vi "Find Average Center.vi"(5 "Position":i32, 7 "Tray Number":i32, 8 "Assembly Type":string, 9 "XYZTheta":dbl[](array[numeric]), 11 "Gantry In":refnum<k24>) -> (1 "XYZTheta":dbl[](array[numeric]) format="%.6g", 3 "Gantry Out":refnum<k24>)   [LabVIEW 2021, in "Component Tray.lvclass"]
uses:
  Component Tray.lvclass
  Find Component.ctl
  Controller/Camera/Machine Vision.ctl
  C:/Program Files (x86)/Aerotech/A3200/LabVIEW/2010/Bin/Aerotech.A3200.dll
  Program Files (x86)/Aerotech/A3200/LabVIEW/2010/Bin/Aerotech.A3200.dll
  Controller/Camera/Image processing.ctl
  Controller/Camera/Camera settings.ctl
  Controller/Camera/Material.ctl
  Controller/Camera/Edmund Optics/Edmund Optics.lvclass
  C:/Users/HEP/Documents/GitHub/Gantry/UCSB-Gantry-HEP-main/Classes/Controller/Camera/Camera.lvclass
  Controller/Camera/Camera.lvclass
  Controller/Motion/A3200/A3200.lvclass
  Controller/Motion/Motion.lvclass
  Routine/TypeOfHexaboard.ctl
  Routine/Routine.lvclass
panel:
  out "Current Z High Speed":dbl
  out "Current XY High Speed":dbl
  out "current Z low speed":dbl
  out "current XY speed":dbl
  in  "Z high":dbl=12.5
  in  "XY high":dbl=50.0
  in  "Z low":dbl=0.05
  in  "XY low":dbl=0.1
  in  "Predict fiducials":bool
  out "Low Speed":bool
  out "X":bool
  out "Y":bool
  out "Z":bool
  out "High Speed":bool
  in  "Go to CH191/FD5":bool
  in  "Go to CH197/FD4":bool
  out "Program Stopped":bool
  out "XY Graph":cluster{"X":dbl, "Y":dbl}[](graph)
  out "Sensor ID Location":dbl[](array[numeric])
  in  "Go to Sensor ID":bool
  out "CH1 Location":dbl[](array[numeric])
  in  "Verify CH1":bool
  out "CH1 correct?":bool
  in  "Go to CH1":bool
  in  "Focus step size":dbl format="%#_13g"
  in  "number of focus steps":i32
  out "Average Strength":dbl
  in  "Focus":bool
  in  "Material":T1
  out "All fiducials recorded":bool
  in  "Override presets":bool
  in  "Camera settings":T2={"Gamma"=1.6, "Gain"=0, "Sharpness"=0, "Contrast"=0.0, "Exposure"=0.0078125} {"Exposure" min=0.000244140625 max=0.5 scale=0.0002..0.5; "Contrast" min=0.0 max=1.0 scale=0.001..1.0; "Sharpness" min=0 max=2 step=1 scale=0.0..2.0; "Gain" min=0 max=100 step=1 scale=0.1..100.0; "Gamma" min=0.01 max=10.0 scale=0.01..10.0}
  in  "Image processing":T3={"Brightness"=128.0, "Contrast"=45.0, "Gamma"=1.0471123} {"Brightness" scale=0.0..400.0; "Contrast" scale=0.0..90.0; "Gamma" scale=0.005..5.0}
  in  "Machine Vision":T4=enum."Sensor Fiducials"
  out "Gantry":dbl[](array[numeric]) format="%.6g"
  out "Sum":dbl[](array[numeric]) format="%.6g"
  out "CH197/FD4 XY":dbl[](array[numeric]) format="%.6g"
  out "CH8/FD2 XY":dbl[](array[numeric]) format="%.6g"
  out "CH191/FD5 XY":dbl[](array[numeric]) format="%.6g"
  out "CH1/FD1 XY":dbl[](array[numeric]) format="%.6g"
  in  "Record CH8/FD2":bool
  in  "Record CH197/FD4":bool
  in  "Record CH191/FD5":bool
  in  "Record CH1/FD1":bool
  in  "Go to CH8/FD2":bool
  in  "Go to CH1/FD1":bool
  in  "Joystick":bool
  out "Camera":dbl[](array[numeric]) format="%.6g"
  in  "Go to Center":bool
  in  "Component":T5
  in  "Stop Program":bool
  out "Image":T6(plugin-control)
  # "Requires CH1/FD1 found."
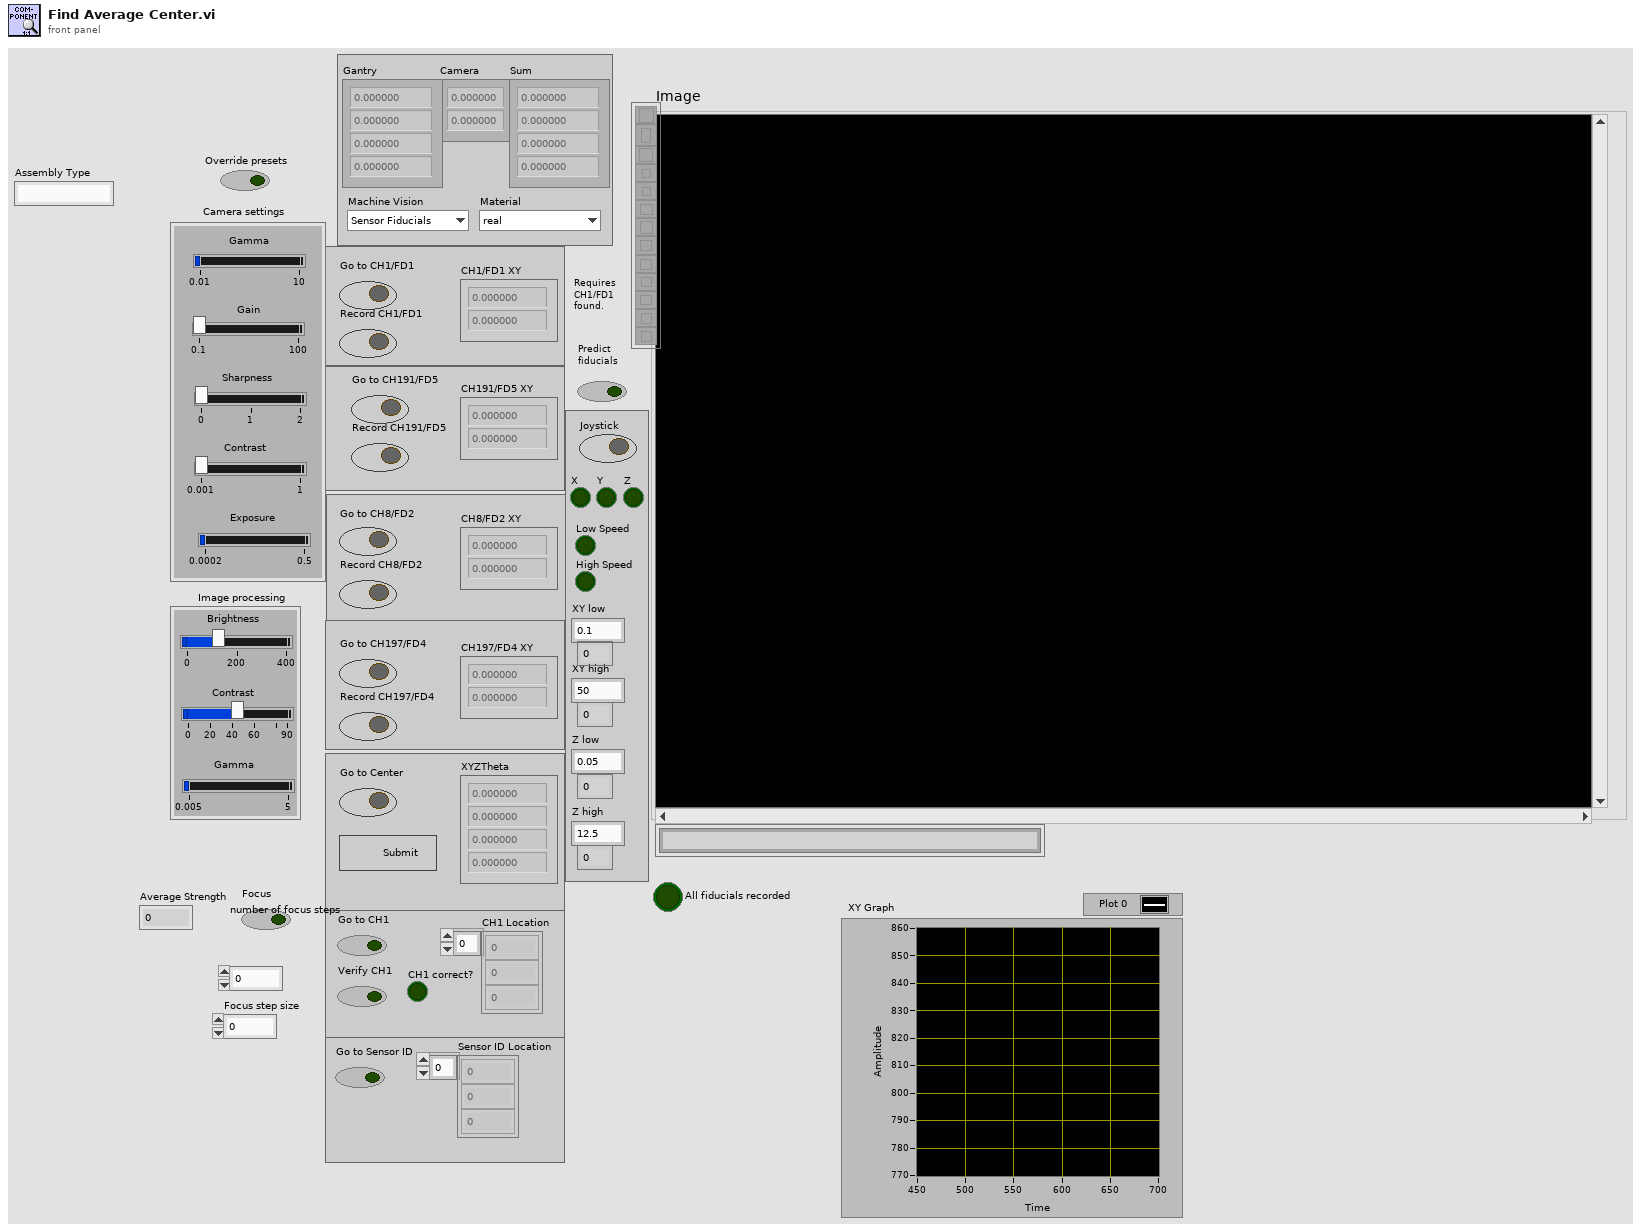
[diagram p1: front panel]
types:
  T1 = typedef "Camera.lvclass/Material.ctl" = enum16{"real", "dummy", "PETG"}
  T2 = typedef "Camera.lvclass/Camera settings.ctl" = cluster{"Gamma":dbl, "Gain":i64, "Sharpness":i64, "Contrast":dbl, "Exposure":dbl}
  T3 = typedef "Camera.lvclass/Image processing.ctl" = cluster{"Brightness":sgl, "Contrast":sgl, "Gamma":sgl}
  T4 = typedef "Camera.lvclass/Machine Vision.ctl" = enum16{"None", "Tray Fiducials", "Sensor Fiducials", "HPK Silicon", "Partial Hexaboard", "Partial Hexaboard Test", "100um dot", "Hexaboard", "Corner (TL, BR)", "Corner (BL, TR)", "V3 Sensor Cross", "V3 Sensor Circle", "test"}
  T5 = typedef "Component Tray.lvclass/Find Component.ctl" = cluster{"New Fiducials":dbl[], "Past Fiducials":dbl[][], "XYZTheta":dbl[], "Fiducials Path":path, "Position":i32, "CH1 Location":dbl[], "Sensor ID Location":dbl[]}
  T6 = typedef "IMAQ Image.ctl" = refnum<image>
  T7 = typedef "Routine.lvclass/TypeOfHexaboard.ctl" = enum16{"Full Sensor", "Full PCB", "Right Partial PCB", "Right Partial Sensor", "Al Dummy Right Partial Sensor"}
  T8 = typedef "File Paths.ctl" = cluster{"Glue Pattern Folder":path, "Carrier Tray Folder":path, "Pick Up Tool Fixture Folder":path, "Components Folder":path, "Bellows Tool Offset.txt":path, "Pick Up Tool Offset.txt":path, "Dispense Tip Offset.txt":path, "Log Files":path, "Gantry Assembly Map.txt":path, "Syringe and offset map.txt":path, "Controllers Folder":path, "Local dbase config":path}
  T9 = enum8{"Enabled", "Disabled", "Disabled and Grayed Out"}
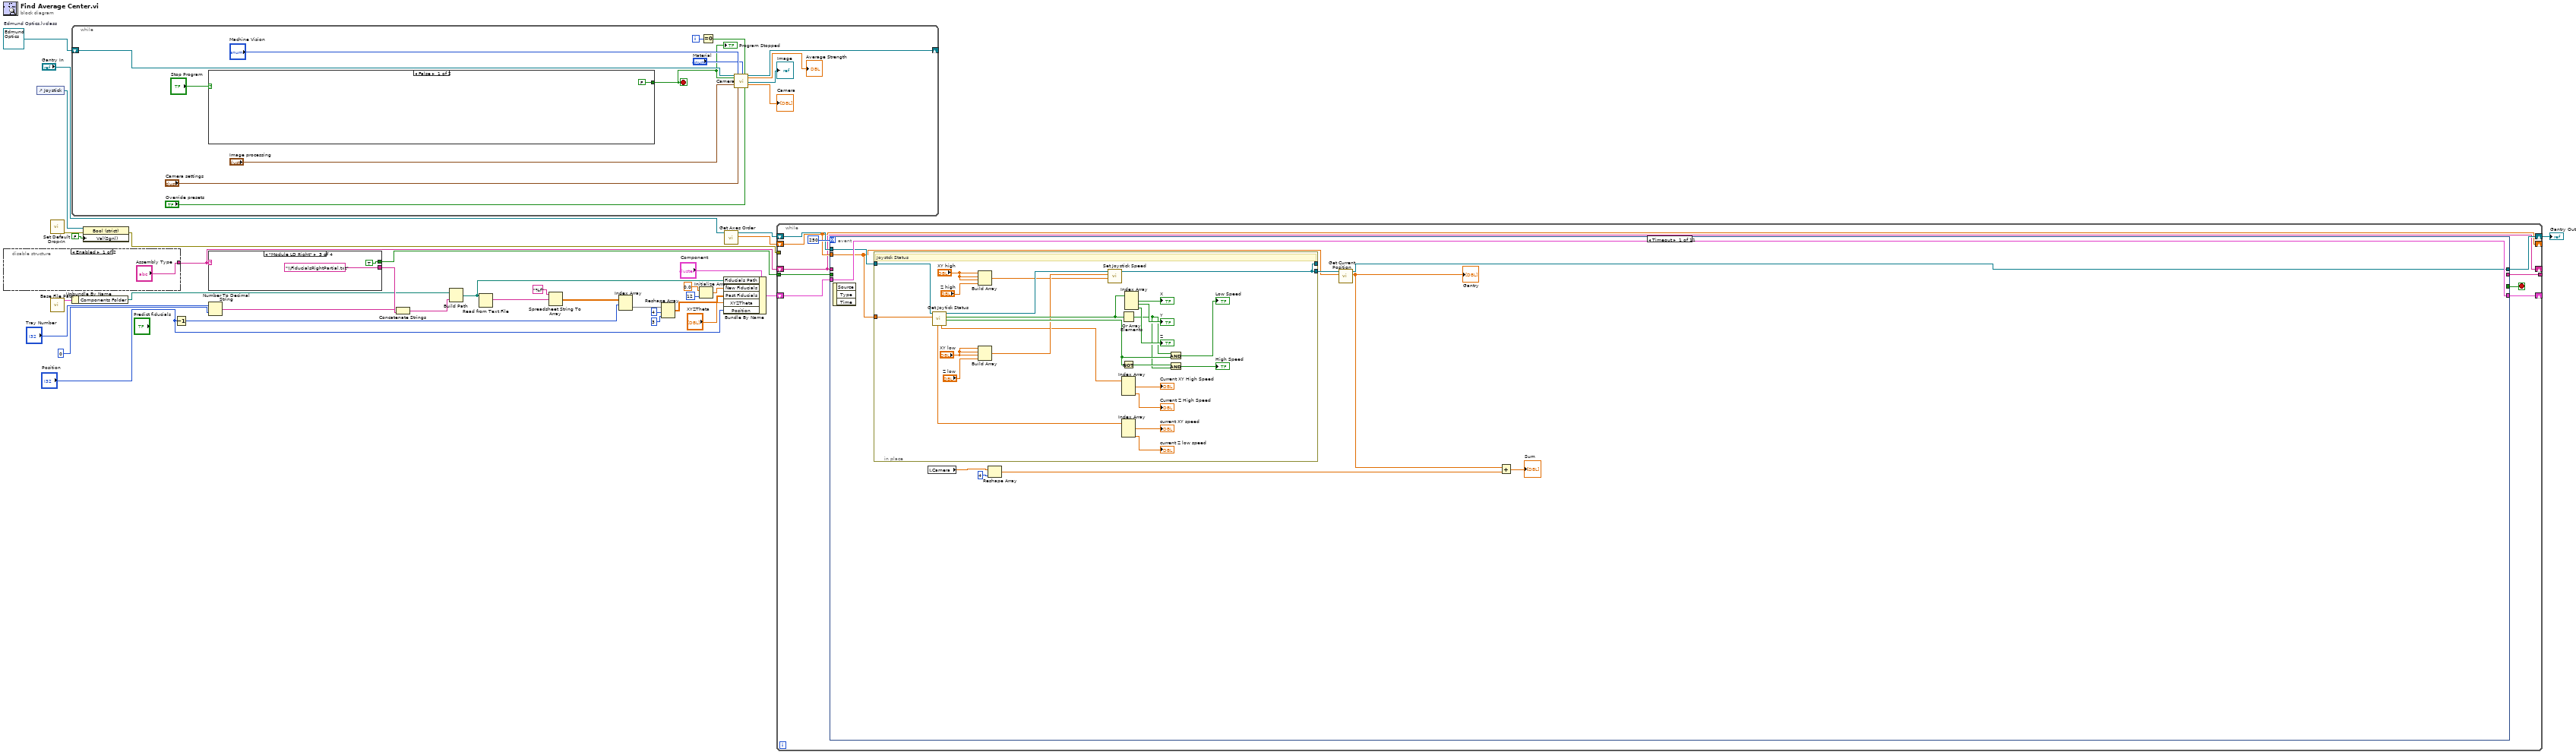
[diagram p0: block diagram]
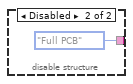
[diagram p2: hidden frame]
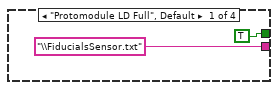
[diagram p3: hidden frame]
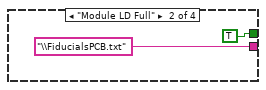
[diagram p4: hidden frame]
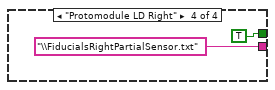
[diagram p5: hidden frame]
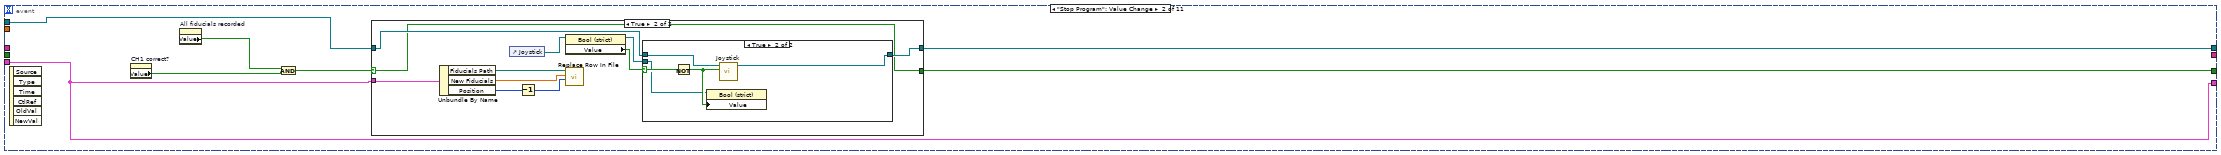
[diagram p6: hidden frame]
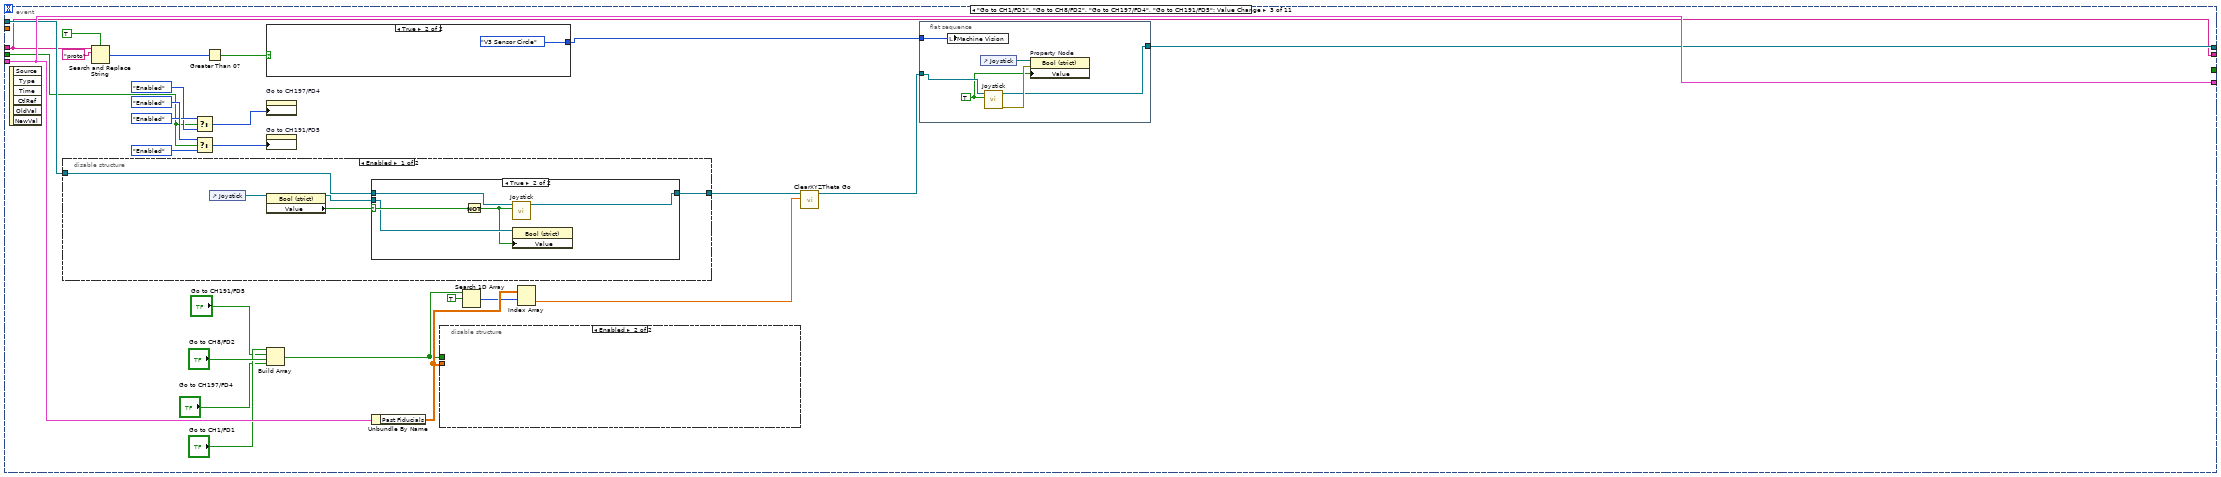
[diagram p9: hidden frame]
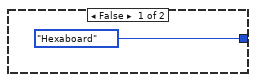
[diagram p10: hidden frame]
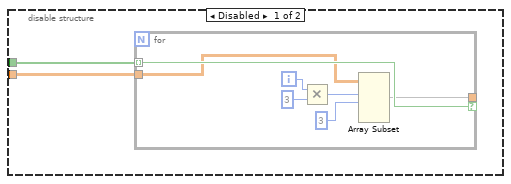
[diagram p11: hidden frame]
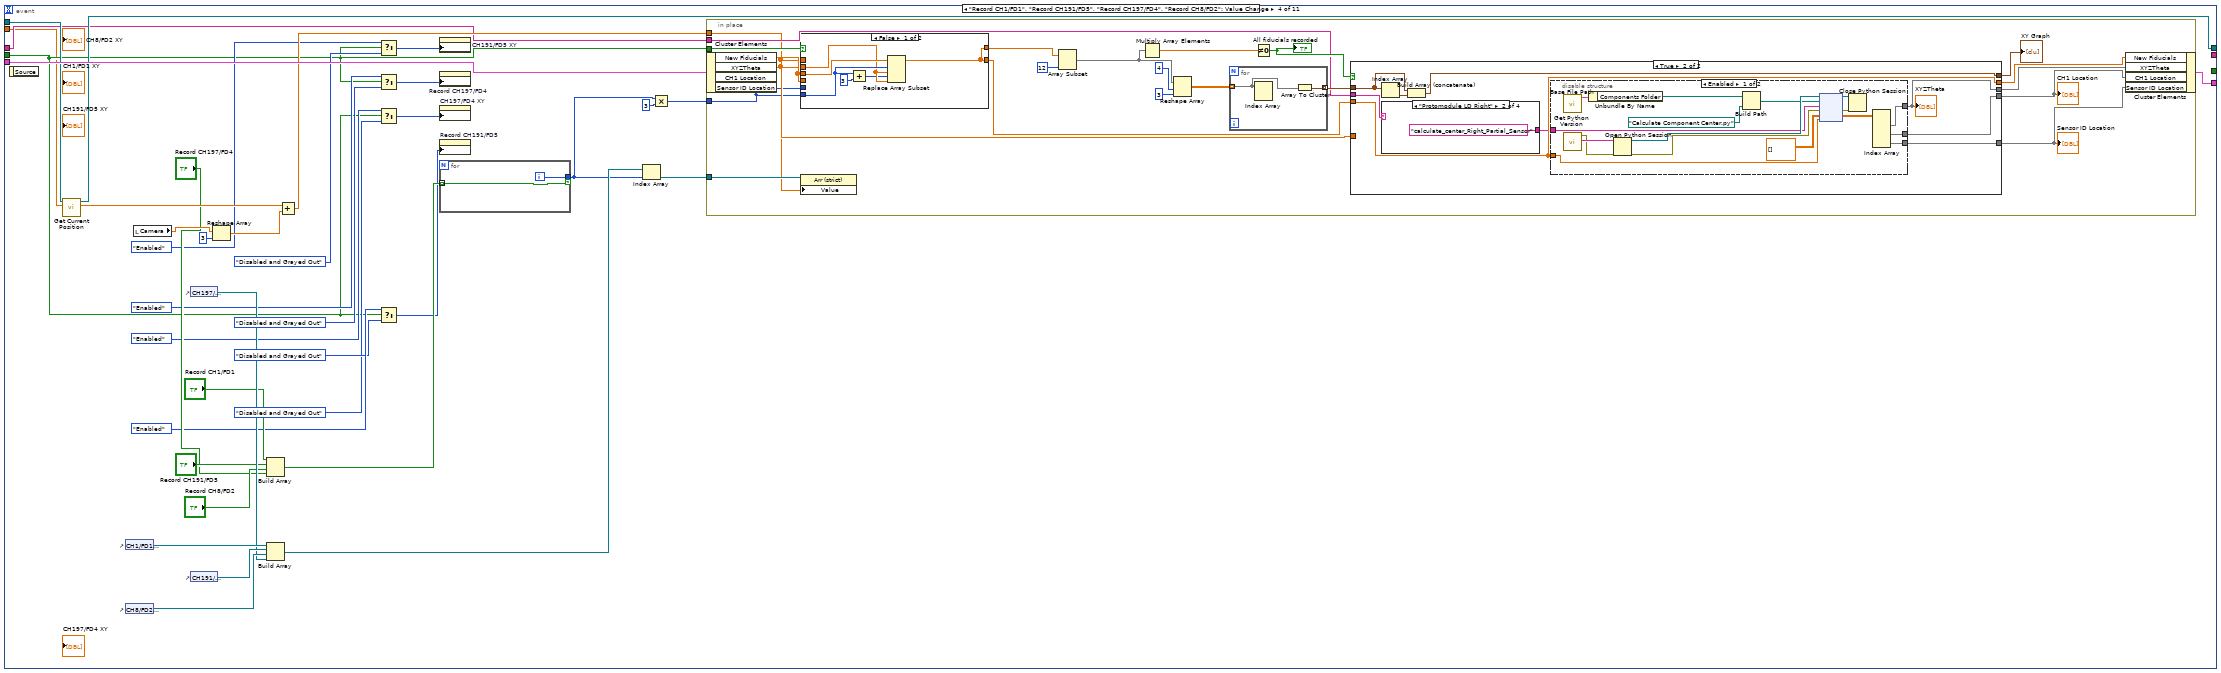
[diagram p14: hidden frame]
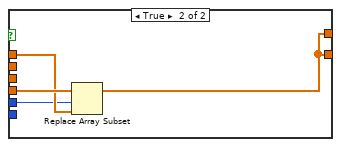
[diagram p15: hidden frame]
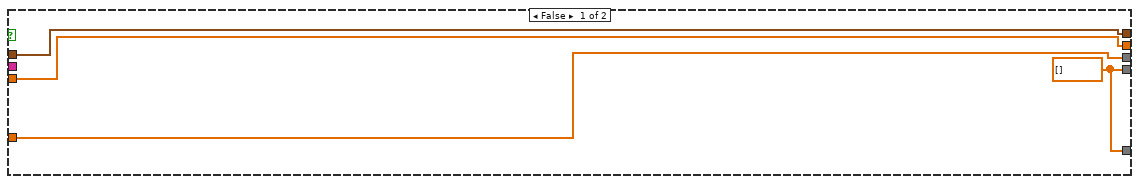
[diagram p16: hidden frame]
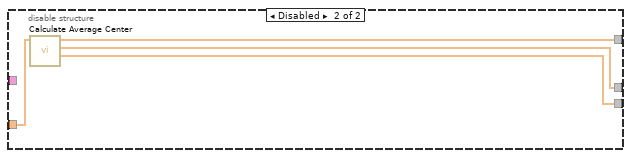
[diagram p17: hidden frame]
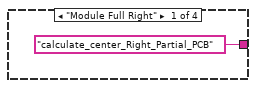
[diagram p18: hidden frame]
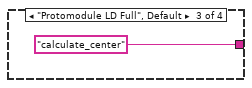
[diagram p19: hidden frame]
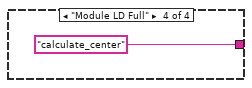
[diagram p20: hidden frame]
diagram:
  w30 = refnum<class "Edmund Optics.lvclass"> refnum  # Edmund Optics.lvclass
  n1 = disable-structure shown="Enabled" {
    disable-tunnel: ["Assembly Type" TypeOfHexaboard."Full PCB" ("Type of Hexaboard")] -> w9
    frame Enabled {
    }
    frame Disabled {
    }
  }
  n2 = control-ref of="Joystick"() -> (w33:refnum<vi>)
  n3 = call "Set Default Drop-In.vi"() -> ("error out"=w12:errorcluster)  [unwired: 11 in]
  n4 = call "Base File Path.vi"() -> ("Paths Out"=w21:T8)  [unwired: 11 in]
  n5 = while {
    shift-right: [w46] -> _
    shift-left: w30 -> [w50]
    i -> [w42]
    stop <- w37 stop-if-true
    n6 = case shown="False" "Stop Program" {
      tunnel: [FALSE w52] -> w37
      frame False {
      }
      frame True {
        n7 = property on="CH1 correct?" class="Bool (strict)"() -> ("Value"=w53:bool)  [unwired: 2 in, 2 out]
        n8 = property on="All fiducials recorded" class="Bool (strict)"() -> ("Value"=w55:bool)  [unwired: 2 in, 2 out]
        n9 = And(x=w55, y=w53) -> (x .and. y?=w54:bool)
        n10 = case shown="False" w54 {
          tunnel: [FALSE TRUE] -> w52
          frame False {
            n11 = One Button Dialog(message="At least one fiducial not recorded or component orientation not verified.") -> ()  [unwired: 1 in, 1 out]
          }
          frame True {
            n12 = property on="All fiducials recorded" class="Bool (strict)"("Val(Sgnl)"=FALSE) -> ()  [unwired: 2 in, 2 out]
          }
        }
      }
    }
    "Program Stopped" <- w37
    n13 = Equal To 0?(x=w42) -> (x = 0?=w41:bool)
    n14 = call "Camera.vi"("Camera in"=w50, "Stop"=w37, "BCG Image Processing"="Image processing", "Machine Vision"="Machine Vision", "Camera settings"="Camera settings", "Material"="Material", "Loop 0"=w41, "Override presets"="Override presets") -> ("Camera out"=w46:refnum<class "Edmund Optics.lvclass">, "Average Strength"=→"Average Strength":dbl, "Image"=→"Image":T6, "Camera"=→"Camera":dbl[])  [unwired: 5 in, 3 out]
  }
  n15 = Unbundle By Name(w21) -> ("Components Folder"=w23:path)
  n16 = property class="Bool (strict)"(reference=w33, error in=w12, "Val(Sgnl)"=FALSE) -> (error out=w31:errorcluster)  [unwired: 1 out]
  n17 = Decrement(x="Position") -> (x-1=w13:i32)
  n18 = case shown="\"Module LD Right\"" w9 {
    tunnel: ["\\FiducialsSensor.txt" ("string") "\\FiducialsPCB.txt" ("string") "\\FiducialsRightPartial.txt" ("string") "\\FiducialsRightPartialSensor.txt" ("string")] -> w25
    tunnel: [TRUE TRUE TRUE TRUE] -> w8
    frame "Protomodule LD Full", Default {
    }
    frame "Module LD Full" {
    }
    frame "Module LD Right" {
    }
    frame "Protomodule LD Right" {
    }
  }
  n19 = Number To Decimal String(number="Tray Number", width (-)=i16 0) -> (decimal integer string=w24:string)
  n20 = Concatenate Strings "Concatenate Strings"(w24, w25) -> (w26:string)
  n21 = Build Path(base path=w23, name or relative path=w26) -> (appended path=w16:path)
  n22 = Read from Text File(file (use dialog)=w16) -> (text=w27:string)  [unwired: 3 in, 3 out]
  n23 = Spreadsheet String To Array(format string="%f", spreadsheet string=w27) -> (array=w29:dbl[][])  [unwired: 2 in]
  n24 = Index Array "Index Array"(array=w29, index (row)=w13) -> (element=w4:dbl[])  [unwired: 1 in]
  n25 = Reshape Array(w4, 4 ("dimension size"), 3 ("dimension size")) -> (w1:dbl[][])
  n26 = Initialize Array(0.0 ("element"), 12 ("dimension size")) -> (w19:dbl[])
  n27 = Bundle By Name "Bundle By Name"(cluster="Component", "Fiducials Path"=w16, "New Fiducials"=w19, "Past Fiducials"=w1, "XYZTheta"="XYZTheta", "Position"="Position") -> (w10:T5)
  n28 = call "Get Axes Order.vi"("Gantry In"="Gantry In") -> ("Axes Order"=w5:dbl[], "Gantry Out"=w6:refnum<k24>)  [unwired: 8 in, 1 out]
  n29 = while {
    shift-right: [w75] -> _
    shift-left: w10 -> [w76]
    tunnel: w31 -> [_]
    shift-right: [w72] -> w11
    shift-left: w6 -> [w73]
    tunnel: [w71] -> _
    tunnel: w8 -> [w70]
    shift-right: [w69] -> _
    shift-left: w5 -> [w69]
    shift-right: [w68] -> _
    shift-left: w9 -> [w68]
    stop <- w77 stop-if-true
    n30 = event shown="[0] Timeout" {
      selector: _ -> [_ _ _ _ _ _ _ _ _ _ _]
      dyn-events: _ -> [_ _ _ _ _ _ _ _ _ _ _]
      timeout: 250 -> [_ _ _ _ _ _ _ _ _ _ _]
      tunnel: [_ w116 _ _ _ _ _ _ _ _ _] -> w77
      tunnel: w76 -> [w86 w118 w165 w231 w317 w355 w403 w410 w425 w440 w450]
      tunnel: [w86 w118 w165 w230 w316 w355 w403 w410 w425 w440 w450] -> w75
      tunnel: w73 -> [w80 w119 w164 w222 w315 w357 w402 w406 w421 w436 w451]
      tunnel: [w82 w117 w161 w220 w315 w356 w400 w404 w419 w434 w451] -> w72
      tunnel: w68 -> [_ _ w141 w219 w311 _ _ _ _ _ _]
      tunnel: [_ _ w141 _ _ _ _ _ _ _ _] -> w71
      tunnel: w70 -> [_ _ w150 w195 _ _ _ _ _ _ _]
      tunnel: w69 -> [w78 _ _ w194 _ w345 _ _ _ _ _]
      event Timeout {
        n31 = event-data() -> ()  [unwired: 1 in, 3 out]
        n32 = in-place {
          in-place-border: w80 -> [w112]
          in-place-border: [w100] -> _
          in-place-border: w78 -> [w111]
          in-place-border: [w100] -> w79
          # "Joystck Status"
          n33 = call "Get Joytick Status.vi"("Axes Order"=w111, "Gantry In"=w112) -> ("JoystickLowSpeedActive"=w105:bool, "Joystick Status"=w107:bool[], "Gantry Out"=w101:refnum<k24>, "High Speeds"=w89:dbl[], "Low Speeds"=w88:dbl[])  [unwired: 4 in, 1 out]
          n34 = Build Array("XY high", "XY high", "XY high", "Z high") -> (w94:dbl[])
          n35 = Build Array("XY low", "XY low", "XY low", "Z low") -> (w95:dbl[])
          n36 = call "Set Joystick Speed.vi"("High Speed Inputs"=w94, "Low Speed Inputs"=w95, "Gantry"=w101) -> ("Controller Out"=w100:refnum<k24>)  [unwired: 7 in, 1 out]
          n37 = Or Array Elements(Boolean array=w107) -> (logical OR=w103:bool)
          n38 = Not(x=w105) -> (.not. x?=w104:bool)
          n39 = Index Array(array=w89) -> (element #1=→"Current XY High Speed":dbl, element #3=→"Current Z High Speed":dbl)  [unwired: 3 in, 1 out]
          n40 = Index Array(array=w88) -> (element #1=→"current XY speed":dbl, element #3=→"current Z low speed":dbl)  [unwired: 3 in, 1 out]
          n41 = Index Array(array=w107) -> (element #1=→"X":bool, element #2=→"Y":bool, element #3=→"Z":bool)  [unwired: 3 in]
          n42 = And(x=w103, y=w105) -> (x .and. y?=→"Low Speed":bool)
          n43 = And(x=w104, y=w103) -> (x .and. y?=→"High Speed":bool)
        }
        n44 = local read "Camera"() -> (w85:dbl[])
        n45 = Reshape Array(w85, 4 ("dimension size")) -> (w83:dbl[])
        n46 = call "Get Current Position.vi"("Axes Order"=w78, "Gantry In"=w79) -> ("XYZTheta Out"=w81:dbl[], "Gantry Out"=w82:refnum<k24>)  [unwired: 7 in, 1 out]
        "Gantry" <- w81
        n47 = Add(x=w81, y=w83) -> (x+y=→"Sum":dbl[])
      }
      event "Stop Program": Value Change {
        n48 = event-data() -> ()  [unwired: 1 in, 6 out]
        n49 = property on="CH1 correct?" class="Bool (strict)"() -> ("Value"=w115:bool)  [unwired: 2 in, 2 out]
        n50 = property on="All fiducials recorded" class="Bool (strict)"() -> ("Value"=w114:bool)  [unwired: 2 in, 2 out]
        n51 = And(x=w114, y=w115) -> (x .and. y?=w113:bool)
        n52 = case shown="True" w113 {
          selector: w113 -> [w120 w129]
          tunnel: w119 -> [w121 w131]
          tunnel: w118 -> [_ w132]
          tunnel: [w121 w130] -> w117
          tunnel: [w120 w129] -> w116
          frame False {
          }
          frame True {
            n53 = Unbundle By Name(w132) -> ("Fiducials Path"=w126:path, "New Fiducials"=w125:dbl[], "Position"=w127:i32)
            n54 = control-ref of="Joystick"() -> (w123:refnum<vi>)
            n55 = Decrement(x=w127) -> (x-1=w128:i32)
            n56 = property class="Bool (strict)"(reference=w123) -> (reference out=w122:refnum<vi>, "Value"=w124:bool)  [unwired: 1 in, 1 out]
            n57 = call "Replace Row In File.vi"("Index"=w128, "Insert Array"=w125, "Path"=w126) -> ()  [unwired: 8 in, 1 out]
            n58 = case shown="True" w124 {
              selector: w124 -> [_ w138]
              tunnel: w131 -> [w133 w137]
              tunnel: [w133 w136] -> w130
              tunnel: w122 -> [_ w134]
              frame False {
              }
              frame True {
                n59 = Not(x=w138) -> (.not. x?=w135:bool)
                n60 = property class="Bool (strict)"(reference=w134, "Value"=w135) -> ()  [unwired: 1 in, 2 out]
                n61 = call "Joystick.vi"("Joystick"=w135, "Gantry In"=w137) -> ("Gantry Out"=w136:refnum<k24>)  [unwired: 8 in, 1 out]
              }
            }
          }
        }
      }
      event "Go to CH1/FD1", "Go to CH8/FD2", "Go to CH197/FD4", "Go to CH191/FD5": Value Change {
        n62 = event-data() -> ()  [unwired: 1 in, 6 out]
        n63 = disable-structure shown="Enabled" {
          disable-tunnel: w164 -> [w179 _]
          disable-tunnel: [w178 _] -> w163
          frame Enabled {
            n64 = control-ref of="Joystick"() -> (w177:refnum<vi>)
            n65 = property class="Bool (strict)"(reference=w177) -> (reference out=w180:refnum<vi>, "Value"=w181:bool)  [unwired: 1 in, 1 out]
            n66 = case shown="True" w181 {
              selector: w181 -> [_ w187]
              tunnel: w179 -> [w182 w185]
              tunnel: [w182 w183] -> w178
              tunnel: w180 -> [_ w186]
              frame False {
              }
              frame True {
                n67 = Not(x=w187) -> (.not. x?=w184:bool)
                n68 = call "Joystick.vi"("Joystick"=w184, "Gantry In"=w185) -> ("Gantry Out"=w183:refnum<k24>)  [unwired: 8 in, 1 out]
                n69 = property class="Bool (strict)"(reference=w186, "Value"=w184) -> ()  [unwired: 1 in, 2 out]
              }
            }
          }
          frame Disabled {
          }
        }
        n70 = Search and Replace String(case sensitive?=TRUE ("ignore case? (F)"), input string=w141, search string="proto") -> (number of replacements=w142:i32)  [unwired: 5 in, 3 out]
        n71 = Select(t=T9."Enabled" ("Disabled"), s=w150, f=T9."Enabled" ("Disabled")) -> (s? t:f=w151:T9)
        n72 = Select(t=T9."Enabled" ("Disabled"), s=w150, f=T9."Enabled" ("Disabled")) -> (s? t:f=w154:T9)
        n73 = Greater Than 0?(x=w142) -> (x > 0?=w139:bool)
        n74 = case shown="True" w139 {
          tunnel: [Machine_Vision."Hexaboard" ("Machine Vision") Machine_Vision."V3 Sensor Circle" ("Machine Vision")] -> w140
          frame False {
          }
          frame True {
          }
        }
        n75 = property on="Go to CH197/FD4" class="Bool"("DisabledEnum"=w151) -> ()  [unwired: 2 in, 2 out]
        n76 = property on="Go to CH191/FD5" class="Bool"("DisabledEnum"=w154) -> ()  [unwired: 2 in, 2 out]
        n77 = Build Array "Build Array"("Go to CH1/FD1", "Go to CH191/FD5", "Go to CH8/FD2", "Go to CH197/FD4") -> (w147:bool[])
        n78 = Unbundle By Name(w165) -> ("Past Fiducials"=w149:dbl[][])
        n79 = disable-structure shown="Enabled" {
          disable-tunnel: w149 -> [w169 _]
          disable-tunnel: w147 -> [w168 _]
          frame Disabled {
            n80 = for {
              tunnel: w168 -> [w176] mode=indexing
              tunnel: w169 -> [w175]
              tunnel: [w170] -> _ if=w176
              i -> [w173]
              n81 = Multiply(x=w173, y=3) -> (x*y=w171:i32)
              n82 = Array Subset "Array Subset"(array=w175, index (row)=w171, length (row)=3 ("length")) -> (w170:dbl[][])  [unwired: 2 in]
            }
          }
          frame Enabled {
          }
        }
        n83 = Search 1D Array(1D array=w147, element=TRUE) -> (index of element=w145:i32)  [unwired: 1 in]
        n84 = Index Array(array=w149, index (row)=w145) -> (element=w148:dbl[])  [unwired: 1 in]
        n85 = call "ClearXYZTheta Go.vi"("XYZTheta In"=w148, "Gantry In"=w163) -> ("Gantry Out"=w162:refnum<k24>)  [unwired: 7 in, 2 out]
        n86 = flat-sequence {
          tunnel: w162 -> [w193]
          tunnel: [w190] -> w161
          tunnel: w140 -> [w188]
          frame #0 {
            w189 = TRUE
            n87 = local write "Machine Vision"(w188) -> ()
            n88 = control-ref of="Joystick"() -> (w192:refnum<vi>)
            n89 = call "Joystick.vi"("Joystick"=w189, "Gantry In"=w193) -> ("error out"=w191:errorcluster, "Gantry Out"=w190:refnum<k24>)  [unwired: 8 in]
            n90 = property on="Property Node" class="Bool (strict)"(reference=w192, error in=w191, "Value"=w189) -> ()  [unwired: 2 out]
          }
        }
      }
      event "Record CH1/FD1", "Record CH191/FD5", "Record CH197/FD4", "Record CH8/FD2": Value Change {
        n91 = event-data() -> ()  [unwired: 1 in, 1 out]
        n92 = call "Get Current Position.vi"("Axes Order"=w194, "Gantry In"=w222) -> ("XYZTheta Out"=w221:dbl[], "Gantry Out"=w220:refnum<k24>)  [unwired: 7 in, 1 out]
        n93 = control-ref of="CH1/FD1 XY"() -> (w217:refnum<vi>)
        n94 = control-ref of="CH8/FD2 XY"() -> (w215:refnum<vi>)
        n95 = local read "Camera"() -> (w225:dbl[])
        n96 = control-ref of="CH197/FD4 XY"() -> (w214:refnum<vi>)
        n97 = control-ref of="CH191/FD5 XY"() -> (w216:refnum<vi>)
        n98 = Reshape Array(w225, 3 ("dimension size")) -> (w224:dbl[])
        n99 = Build Array "Build Array"("Record CH1/FD1", "Record CH191/FD5", "Record CH8/FD2", "Record CH197/FD4") -> (w218:bool[])
        n100 = Build Array "Build Array"(w217, w216, w215, w214) -> (w229:refnum<vi>[])
        n101 = Add(x=w221, y=w224) -> (x+y=w223:dbl[])
        n102 = Select(t=T9."Enabled" ("Disabled"), s=w195, f=T9."Disabled and Grayed Out" ("Disabled")) -> (s? t:f=w200:T9)
        n103 = Select(t=T9."Enabled" ("Disabled"), s=w195, f=T9."Disabled and Grayed Out") -> (s? t:f=w204:T9)
        n104 = Select(t=T9."Enabled" ("Disabled"), s=w195, f=T9."Disabled and Grayed Out" ("Disabled")) -> (s? t:f=w196:T9)
        n105 = Select(t=T9."Enabled" ("Disabled"), s=w195, f=T9."Disabled and Grayed Out") -> (s? t:f=w206:T9)
        n106 = property on="CH191/FD5 XY" class="Arr (strict)"("DisabledEnum"=w200) -> ()  [unwired: 2 in, 2 out]
        n107 = property on="Record CH197/FD4" class="Bool"("DisabledEnum"=w204) -> ()  [unwired: 2 in, 2 out]
        n108 = property on="CH197/FD4 XY" class="Arr (strict)"("DisabledEnum"=w196) -> ()  [unwired: 2 in, 2 out]
        n109 = property on="Record CH191/FD5" class="Bool"("DisabledEnum"=w206) -> ()  [unwired: 2 in, 2 out]
        n110 = for {
          tunnel: w218 -> [w232] mode=indexing
          tunnel: [w233] -> w209 if=w232
          i -> [w233]
        }
        n111 = Index Array "Index Array"(array=w229, index=w209) -> (element=w228:refnum<vi>)
        n112 = Multiply(x=w209, y=3) -> (x*y=w226:i32)
        n113 = in-place {
          in-place-border: w226 -> [w235]
          in-place-border: w228 -> [w253]
          in-place-border: w223 -> [w236]
          in-place-border: w219 -> [w240]
          in-place-border: w195 -> [w238]
          n114 = in-place-cluster #1(w231) -> ("New Fiducials"=w237:dbl[], "XYZTheta"=w252:dbl[])  [unwired: 2 out]
          n115 = case shown="False" w238 {
            tunnel: w237 -> [w261 _]
            tunnel: w235 -> [w260 _]
            tunnel: w236 -> [w259 _]
            tunnel: [w256 w262] -> w239
            tunnel: w237 -> [_ w265]
            tunnel: w236 -> [_ w264]
            tunnel: w235 -> [_ w263]
            tunnel: [w256 w262] -> w234
            frame False {
              n116 = Add(x=w260, y=3) -> (x+y=w257:i32)
              n117 = Replace Array Subset "Replace Array Subset"(array=w261, new element #1=w259, index #1=w260, new element #2=w259, index #2=w257) -> (w256:dbl[])
            }
            frame True {
              n118 = Replace Array Subset "Replace Array Subset"(array=w265, new element=w264, index=w263) -> (w262:dbl[])
            }
          }
          n119 = property class="Arr (strict)"(reference=w253, "Value"=w236) -> ()  [unwired: 1 in, 2 out]
          n120 = Array Subset "Array Subset"(array=w234, length=12) -> (w247:dbl[])  [unwired: 1 in]
          n121 = Multiply Array Elements(1:w247) -> (0:w250:dbl)
          n122 = Reshape Array "Reshape Array"(w247, 4 ("dimension size"), 3 ("dimension size")) -> (w244:dbl[][])
          n123 = for {
            tunnel: w244 -> [w266] mode=indexing
            tunnel: [w267] -> w243 mode=indexing
            n124 = Index Array(array=w266) -> ()  [unwired: 2 in, 2 out]
            n125 = Array To Cluster(array=w266) -> (cluster=w267:cluster{"[0]":dbl, "[1]":dbl})
          }
          n126 = Not Equal To 0?(x=w250) -> (x != 0?=w241:bool)
          "All fiducials recorded" <- w241
          n127 = case shown="True" w241 {
            tunnel: [w270 w273] -> w255
            tunnel: w239 -> [w271 w277]
            tunnel: [w271 w277] -> w254
            tunnel: w252 -> [w270 _]
            tunnel: [w269 w274] -> w249
            tunnel: [w269 w275] -> w248
            tunnel: w243 -> [w268 w280]
            tunnel: [w268 w278] -> w242
            tunnel: w240 -> [_ w276]
            frame False {
              w269 = dbl[] [] ("CH1 location")
            }
            frame True {
              n128 = Index Array(array=w280) -> (element=w279:cluster{"[0]":dbl, "[1]":dbl})  [unwired: 1 in]
              n129 = case shown="\"Protomodule LD Right\"" w276 {
                tunnel: ["calculate_center_Right_Partial_PCB" ("function name") "calculate_center_Right_Partial_Sensor" ("function name") "calculate_center" ("function name") "calculate_center" ("function name")] -> w272
                frame "Module Full Right" {
                }
                frame "Protomodule LD Right" {
                }
                frame "Protomodule LD Full", Default {
                }
                frame "Module LD Full" {
                }
              }
              n130 = Build Array (concatenate)(w280, w279) -> (w278:cluster{"[0]":dbl, "[1]":dbl}[])
              n131 = disable-structure shown="Enabled" {
                disable-tunnel: w277 -> [w288 w298]
                disable-tunnel: [w284 w301] -> w275
                disable-tunnel: [w285 w300] -> w274
                disable-tunnel: [w286 w299] -> w273
                disable-tunnel: w272 -> [w283 _]
                frame Enabled {
                  n132 = call "Base File Path.vi"() -> ("Paths Out"=w293:T8)  [unwired: 11 in]
                  n133 = call "Get Python Version.vi"() -> ("Python Version"=w282:string, "error out"=w281:errorcluster)  [unwired: 10 in]
                  n134 = Unbundle By Name(w293) -> ("Components Folder"=w291:path)
                  n135 = Open Python Session(python version=w282, 3:w281) -> (session out=w297:refnum<k35>, error out=w295:errorcluster)  [unwired: 1 in]
                  n136 = Build Path(base path=w291, name or relative path=path "Calculate Component Center.py") -> (appended path=w290:path)
                  n137 = node(w297, w290, w283, w295, dbl[][] [], w288) -> (w296:refnum<k35>, w294:errorcluster, w287:dbl[][])  [unwired: 1 in, 2 out]
                  n138 = Close Python Session(session in=w296, error in=w294) -> ()  [unwired: 1 out]
                  n139 = Index Array(array=w287) -> (element #1=w286:dbl[], element #2=w285:dbl[], element #3=w284:dbl[])  [unwired: 6 in]
                }
                frame Disabled {
                  n140 = call "Calculate Average Center.vi"("Gantry Fiducials"=w298) -> ("Sensor ID Location"=w301:dbl[], "CH1 Location"=w300:dbl[], "XYZTheta"=w299:dbl[])  [unwired: 8 in]
                }
              }
              "XYZTheta" <- w273
            }
          }
          "CH1 Location" <- w249
          "Sensor ID Location" <- w248
          "XY Graph" <- w242
          n141 = in-place-cluster #1("New Fiducials"=w254, "XYZTheta"=w255, "CH1 Location"=w249, "Sensor ID Location"=w248) -> (w230:T5)
        }
      }
      event "Predict fiducials": Value Change {
        n142 = event-data() -> ()  [unwired: 1 in, 6 out]
        n143 = Unbundle By Name(w317) -> ("New Fiducials"=w336:dbl[], "Position"=w332:i32)  [unwired: 1 out]
        n144 = Search and Replace String(case sensitive?=TRUE ("ignore case? (F)"), input string=w311, search string="proto") -> (number of replacements=w308:i32)  [unwired: 5 in, 3 out]
        n145 = Reshape Array(w336, 4 ("dimension size"), 3 ("dimension size")) -> (w333:dbl[][])
        n146 = Greater Than 0?(x=w308) -> (x > 0?=w307:bool)
        n147 = case shown="False" w307 {
          tunnel: [dbl[] [-160.0, 70.0] ("x") dbl[] [-165.98, 75.999] ("x")] -> w306
          frame False {
          }
          frame True {
          }
        }
        n148 = Equal?(x=w332, y=1) -> (x = y?=w330:bool)
        n149 = case shown="False" w330 {
          tunnel: w306 -> [w342 w344]
          tunnel: [w342 w343] -> w329
          frame False {
          }
          frame True {
            n150 = Negate(x=w344) -> (-x=w343:dbl[])
          }
        }
        n151 = Index Array(array=w329) -> (element #1=w324:dbl, element #2=w323:dbl)  [unwired: 2 in]
        n152 = Build Array(w324, 0.0 ("element"), 0.0 ("element")) -> (w325:dbl[])
        n153 = Build Array(w324, w323, 0.0 ("element")) -> (w322:dbl[])
        n154 = Build Array(0.0 ("element"), w323, 0.0 ("element")) -> (w326:dbl[])
        n155 = Build Array(w325, w326, w322) -> (w321:dbl[][])
        n156 = Index Array(array=w333) -> (element=w320:dbl[])  [unwired: 2 in]
        n157 = for {
          tunnel: w321 -> [w341] mode=indexing
          tunnel: w320 -> [w340]
          tunnel: [w339] -> w319 mode=indexing
          n158 = Add(x=w341, y=w340) -> (x+y=w339:dbl[])
        }
        n159 = Build Array (concatenate)(w320, w319) -> (w318:dbl[][])
        n160 = Bundle By Name(cluster=w317, "Past Fiducials"=w318) -> (w316:T5)
      }
      event "Focus": Value Change {
        n161 = event-data() -> ()  [unwired: 1 in, 6 out]
        n162 = Divide(x="number of focus steps", y=2) -> (x/y=w360:dbl)
        n163 = Multiply(x=w360, y="Focus step size") -> (x*y=w358:dbl)
        n164 = call "Joystick.vi"("Joystick"=FALSE, "Gantry In"=w357) -> ("Gantry Out"=w351:refnum<k24>)  [unwired: 8 in, 1 out]
        n165 = Negate(x=w358) -> (-x=w352:dbl)
        n166 = call "Z Go.vi"("Increment"=TRUE, "Return Immediately"=FALSE ("Increment"), "Speed In"=1.0 ("Speed"), "Position In"=w352, "Gantry In"=w351) -> ("error out"=w349:errorcluster, "Gantry Out"=w350:refnum<k24>)  [unwired: 3 in, 2 out]
        n167 = for {
          N: "number of focus steps" -> [_]
          tunnel: [w378] -> w371 mode=indexing
          tunnel: w349 -> [w377]
          tunnel: [w375] -> w364
          shift-right: [w379] -> w365
          shift-left: w350 -> [w381]
          tunnel: "Focus step size" -> [w374]
          tunnel: w345 -> [w373]
          n168 = flat-sequence {
            tunnel: w381 -> [w389]
            tunnel: [w388] -> w380
            tunnel: w377 -> [w387]
            tunnel: [w386] -> w376
            tunnel: w374 -> [w384]
            tunnel: w380 -> [w399]
            tunnel: [w398] -> w379
            tunnel: [w397] -> w378
            tunnel: w376 -> [w393]
            tunnel: [w392] -> w375
            tunnel: w373 -> [w390]
            frame #0 {
              n169 = call "Z Go.vi"("Increment"=TRUE, "Return Immediately"=FALSE ("Increment"), "error in (no error)"=w387, "Speed In"=0.1 ("Speed"), "Position In"=w384, "Gantry In"=w389) -> ("error out"=w386:errorcluster, "Gantry Out"=w388:refnum<k24>)  [unwired: 2 in, 2 out]
            }
            frame #1 {
              n170 = call "Get Current Position.vi"("error in (no error)"=w393, "Axes Order"=w390, "Gantry In"=w399) -> ("error out"=w392:errorcluster, "XYZTheta Out"=w396:dbl[], "Gantry Out"=w398:refnum<k24>)  [unwired: 6 in]
              n171 = local read "Average Strength"() -> (w391:dbl)
              n172 = Delete From Array(array=w396, index=2) -> (deleted portion=w394:dbl)  [unwired: 1 in, 1 out]
              n173 = Build Array(w391, w394) -> (w397:dbl[])
            }
          }
        }
        n174 = Transpose 2D Array(2D array=w371) -> (transposed array=w370:dbl[][])
        n175 = Index Array(array=w370) -> (element #2=w369:dbl[])  [unwired: 4 in, 1 out]
        n176 = Index Array(array=w370) -> (element=w372:dbl[])  [unwired: 2 in]
        n177 = Array Max & Min(array=w372) -> (max index (indices)=w368:i32)  [unwired: 3 out]
        n178 = Index Array(array=w369, index=w368) -> (element=w367:dbl)
        n179 = call "Z Go.vi"("Increment"=FALSE, "Return Immediately"=FALSE ("Increment"), "error in (no error)"=w364, "Speed In"=15.0 ("Speed"), "Position In"=w367, "Gantry In"=w365) -> ("Gantry Out"=w356:refnum<k24>)  [unwired: 2 in, 3 out]
      }
      event "Joystick": Value Change {
        n180 = event-data() -> ()  [unwired: 1 in, 6 out]
        n181 = call "Joystick.vi"("Joystick"="Joystick", "Gantry In"=w402) -> ("Gantry Out"=w400:refnum<k24>)  [unwired: 8 in, 1 out]
      }
      event "Go to Center": Value Change {
        n182 = event-data() -> ()  [unwired: 1 in, 6 out]
        n183 = Unbundle By Name(w410) -> ("XYZTheta"=w411:dbl[])
        n184 = control-ref of="Joystick"() -> (w407:refnum<vi>)
        n185 = property class="Bool (strict)"(reference=w407) -> (reference out=w408:refnum<vi>, "Value"=w409:bool)  [unwired: 1 in, 1 out]
        n186 = case shown="True" w409 {
          selector: w409 -> [_ w418]
          tunnel: w406 -> [w412 w415]
          tunnel: [w412 w414] -> w405
          tunnel: w408 -> [_ w417]
          frame False {
          }
          frame True {
            n187 = Not(x=w418) -> (.not. x?=w413:bool)
            n188 = call "Joystick.vi"("Joystick"=w413, "Gantry In"=w415) -> ("error out"=w416:errorcluster, "Gantry Out"=w414:refnum<k24>)  [unwired: 8 in]
            n189 = property class="Bool (strict)"(reference=w417, error in=w416, "Value"=w413) -> ()  [unwired: 2 out]
          }
        }
        n190 = call "ClearXYZTheta Go.vi"("XYZTheta In"=w411, "Gantry In"=w405) -> ("Gantry Out"=w404:refnum<k24>)  [unwired: 7 in, 2 out]
      }
      event "Go to CH1": Value Change {
        n191 = event-data() -> ()  [unwired: 1 in, 6 out]
        n192 = Unbundle By Name(w425) -> ("CH1 Location"=w426:dbl[])
        n193 = control-ref of="Joystick"() -> (w422:refnum<vi>)
        n194 = property class="Bool (strict)"(reference=w422) -> (reference out=w423:refnum<vi>, "Value"=w424:bool)  [unwired: 1 in, 1 out]
        n195 = case shown="True" w424 {
          selector: w424 -> [_ w433]
          tunnel: w421 -> [w427 w430]
          tunnel: [w427 w429] -> w420
          tunnel: w423 -> [_ w432]
          frame False {
          }
          frame True {
            n196 = Not(x=w433) -> (.not. x?=w428:bool)
            n197 = call "Joystick.vi"("Joystick"=w428, "Gantry In"=w430) -> ("error out"=w431:errorcluster, "Gantry Out"=w429:refnum<k24>)  [unwired: 8 in]
            n198 = property class="Bool (strict)"(reference=w432, error in=w431, "Value"=w428) -> ()  [unwired: 2 out]
          }
        }
        n199 = call "ClearXYZTheta Go.vi"("XYZTheta In"=w426, "Gantry In"=w420) -> ("Gantry Out"=w419:refnum<k24>)  [unwired: 7 in, 2 out]
      }
      event "Go to Sensor ID": Value Change {
        n200 = event-data() -> ()  [unwired: 1 in, 6 out]
        n201 = Unbundle By Name(w440) -> ("Sensor ID Location"=w441:dbl[])
        n202 = control-ref of="Joystick"() -> (w437:refnum<vi>)
        n203 = property class="Bool (strict)"(reference=w437) -> (reference out=w438:refnum<vi>, "Value"=w439:bool)  [unwired: 1 in, 1 out]
        n204 = case shown="True" w439 {
          selector: w439 -> [_ w448]
          tunnel: w436 -> [w442 w445]
          tunnel: [w442 w444] -> w435
          tunnel: w438 -> [_ w447]
          frame False {
          }
          frame True {
            n205 = Not(x=w448) -> (.not. x?=w443:bool)
            n206 = call "Joystick.vi"("Joystick"=w443, "Gantry In"=w445) -> ("error out"=w446:errorcluster, "Gantry Out"=w444:refnum<k24>)  [unwired: 8 in]
            n207 = property class="Bool (strict)"(reference=w447, error in=w446, "Value"=w443) -> ()  [unwired: 2 out]
          }
        }
        n208 = call "ClearXYZTheta Go.vi"("XYZTheta In"=w441, "Gantry In"=w435) -> ("Gantry Out"=w434:refnum<k24>)  [unwired: 7 in, 2 out]
      }
      event "Verify CH1": Value Change {
        n209 = event-data() -> ()  [unwired: 1 in, 6 out]
        "CH1 correct?" <- TRUE
      }
    }
  }
  "Gantry Out" <- w11
